vi "Set_Shortcut.vi"(8 "error in (no error)":errorcluster, 10 "data":T1, 11 "Class in":refnum<class "IB_Shortcut.lvclass">) -> (0 "error out":errorcluster, 3 "Class out":refnum<class "IB_Shortcut.lvclass">)   [LabVIEW 2020, in "IB_Shortcut.lvclass"]
uses:
  <vilib>/AppBuilder/IB_Classes/Shortcut/IB_Shortcut.lvclass
  <vilib>/AppBuilder/IB_Classes/Shortcut/IB_Shortcut.lvclass/IB_Shortcut.ctl
  <vilib>/AppBuilder/IB_Classes/Shortcut/IB_Shortcut.ctl
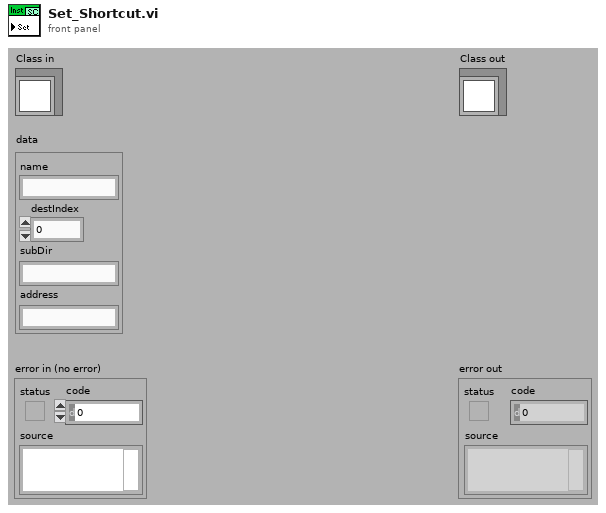
[diagram p1: front panel]
types:
  T1 = typedef "IB_Shortcut.ctl" = cluster{"name":string, "destIndex":i32, "subDir":string, "address":string}
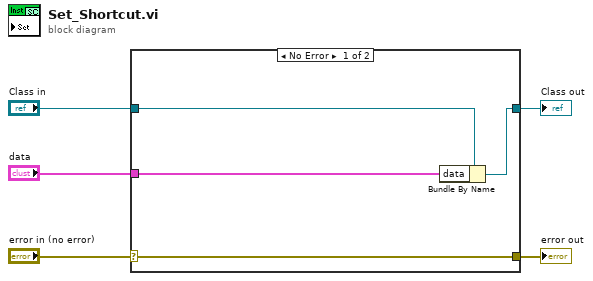
[diagram p0: block diagram]
diagram:
  n1 = case shown="No Error" "error in (no error)" {
    selector: "error in (no error)" -> [w9 w10]
    tunnel: [w9 w10] -> w4
    tunnel: [w7 w11] -> w2
    tunnel: "Class in" -> [w8 w11]
    tunnel: "data" -> [w6 _]
    frame No Error {
      n2 = Bundle By Name(cluster=w8, "data"=w6) -> (w7:refnum<class "IB_Shortcut.lvclass">)
    }
    frame Error {
    }
  }
  "error out" <- w4
  "Class out" <- w2
